vi "RegisterBindingForInstanceSubscriber.vi"(8 "error in (no error)":errorcluster, 10 "binding parameters":string[](array[string]), 11 "service in":refnum<class "IcmMessageService.lvclass">) -> (0 "error out":errorcluster, 3 "service out":refnum<class "IcmMessageService.lvclass">)   [LabVIEW 2017, in "IcmMessageService.lvclass"]
doc: "Registers a message with particular binding parameters."
uses:
  <vilib>/addons/InsightCM/MessageBus/MessageService/IcmMessageService.lvclass
  <vilib>/addons/InsightCM/MessageBus/MessageService/IcmMessageService.lvclass/IcmMessageService.ctl
  C:/Program Files (x86)/National Instruments/LabVIEW 2017/vi.lib/addons/InsightCM/Binaries/LabviewMessageAdapter.dll
  Binaries/LabviewMessageAdapter.dll
  C:/Program Files (x86)/National Instruments/LabVIEW 2017/vi.lib/addons/InsightCM/Binaries/NationalInstruments.MessageBus.dll
  Binaries/NationalInstruments.MessageBus.dll
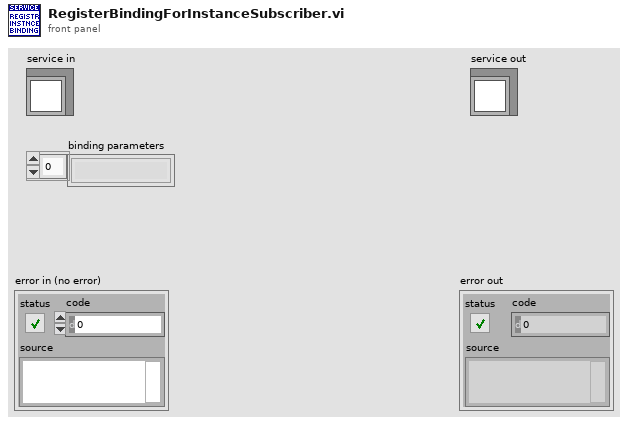
[diagram p1: front panel]
types:
  T1 = typedef "MessageServiceDvr.ctl" = refnum<data-value>
  T2 = typedef "MessageServiceData.ctl" = cluster{"Service":refnum<k24>}
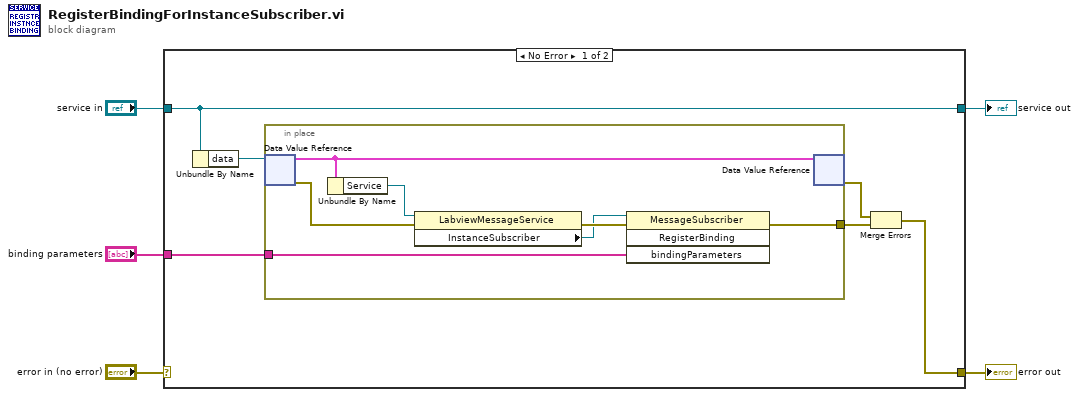
[diagram p0: block diagram]
diagram:
  n1 = case shown="No Error" "error in (no error)" {
    selector: "error in (no error)" -> [_ w20]
    tunnel: [w7 w20] -> w5
    tunnel: [w11 w19] -> w3
    tunnel: "service in" -> [w11 w19]
    tunnel: "binding parameters" -> [w6 _]
    frame No Error {
      n2 = Unbundle By Name(w11) -> ("data"=w10:T1)
      n3 = in-place {
        in-place-border: [w17] -> w8
        in-place-border: w6 -> [w16]
        n4 = in-place-dvr #1(w10) -> (w18:T2, w15:errorcluster)
        n5 = Unbundle By Name(w18) -> ("Service"=w13:refnum<k24>)
        n6 = property class="LabviewMessageService"(reference=w13, error in=w15) -> (error out=w14:errorcluster, "InstanceSubscriber"=w12:refnum<k24>)  [unwired: 1 out]
        n7 = invoke class="MessageSubscriber" method="RegisterBinding"(reference=w12, error in=w14, "bindingParameters"=w16) -> (error out=w17:errorcluster)  [unwired: 1 in, 3 out]
        n8 = in-place-dvr #1(w18) -> (w9:errorcluster)  [unwired: 1 out]
      }
      n9 = Merge Errors(w9, w8) -> (w7:errorcluster)
    }
    frame Error {
    }
  }
  "error out" <- w5
  "service out" <- w3
